vi "Circle Area Perimeter.vi"() -> ()   [LabVIEW 2024]
panel:
  out "Perimeter":dbl
  out "Area":dbl
  in  "r":dbl
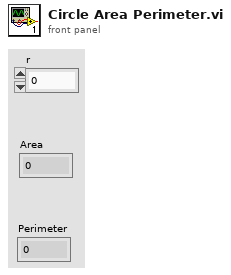
[diagram p1: front panel]
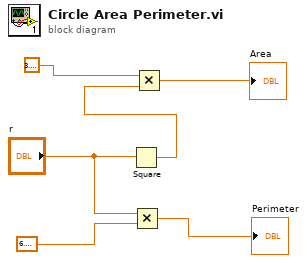
[diagram p0: block diagram]
diagram:
  n1 = Square(x="r") -> (x^2=w2:dbl)
  n2 = Multiply(x="r", y=6.283185307179586) -> (x*y=→"Perimeter":dbl)
  n3 = Multiply(x=3.141592653589793, y=w2) -> (x*y=→"Area":dbl)
